vi "Custom Gauge XControl Demo.vi"() -> ()   [LabVIEW 2012]
doc: "The VI demonstrates how to use a custom XControl that automatically updates the scale of a gauge indicator based on the scaling settings of an existing Shared Variable.\n\nThe source code for the custom XControl can be found in the Auto Scaling Gauge.lvproj example."
uses:
  AutoScalingGauge/CustomGauge.xctl
panel:
  out "String":string="Instructions:\n\nThe gauge indicator below is actually a custom XControl that extends the basic LabVIEW gauge control.\nOpen the project Auto Scaling Gauge.lvproj in the examples folder to see how the XControl was constructed.\n\nThe custom gauge below implements a special right-click menu feature that allows you to quickly bind the gauge to a published shared variable.  Right-click the gauge and choose \"Select Variable...\" to make your selection.  If the variable that you choose has scaling enabled the gauge scale will automatically update with the scaling properties of that variable.\n\nRun the VI after you have selected a variable.  Notice that the gauge is bound to the variable and the label has updated automatically.  Click \"Stop\" or the Abort button to stop the VI."
  in  "?":dbl(xcontrol)
  in  "stop":bool
  # "DSC Module Example Program\nCustom Gauge XControl"
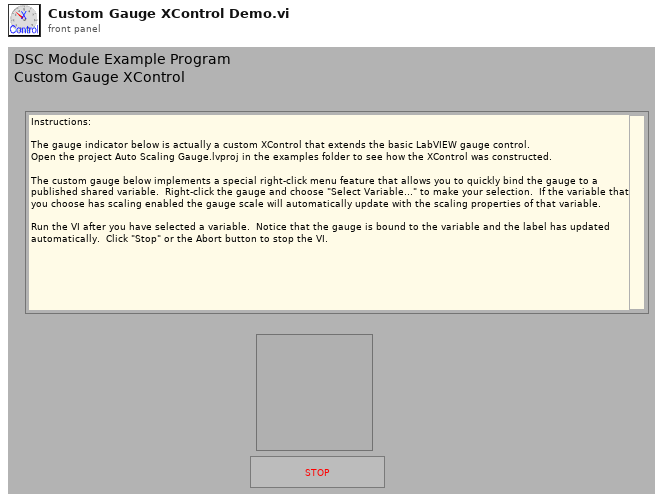
[diagram p1: front panel]
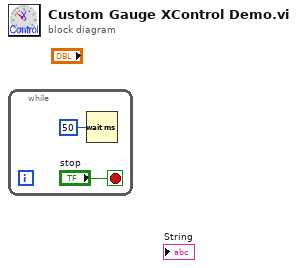
[diagram p0: block diagram]
diagram:
  n1 = while {
    stop <- "stop" stop-if-true
    n2 = Wait (ms)(milliseconds to wait=u32 50) -> ()  [unwired: 1 out]
  }
